vi "stimulate_and_record_async_daq.vi"(3 "SSH password":string, 4 "Transfer and Run Date Folder After Experiment":bool, 5 "SSH user name":string, 6 "Tags":string, 7 "Frames":i32, 8 "Convert Power to Voltage":bool, 9 "voltages/power":dbl[](array[numeric]), 10 "parameters":string[](array[string]), 11 "parameters headers":string[](array[string])) -> ()   [LabVIEW 2016]
uses:
  <vilib>/vision/driver/IMAQdx.llb/IMAQdx Acquisition Mode.ctl
  <vilib>/userdefined/High Color/IMAQdx.ctl
  <vilib>/vision/driver/IMAQdx.llb/IMAQdx Buffer Number Mode.ctl
  <vilib>/Utility/file.llb/Write To Spreadsheet File (DBL).vi
  <vilib>/Utility/file.llb/Write To Spreadsheet File (string).vi
  <vilib>/Utility/file.llb/Read From Spreadsheet File (string).vi
  <vilib>/vision/driver/NI_Vision_Acquisition_Software.lvlib
panel:
  out "DAC0 Voltage":dbl format="%.6f"
  out "error out 2":errorcluster
  out "Saved Buffer Number":u32
  out "ProcessFrameRate":dbl
  out "# elements in queue":i32
  out "CameraFrameRate":dbl
  out "Camera Buffer Number":u32
  out "Image":T1(plugin-control)
  out "JPEG Quality":dbl
  out "Save Directory":path
  in  "stop":bool
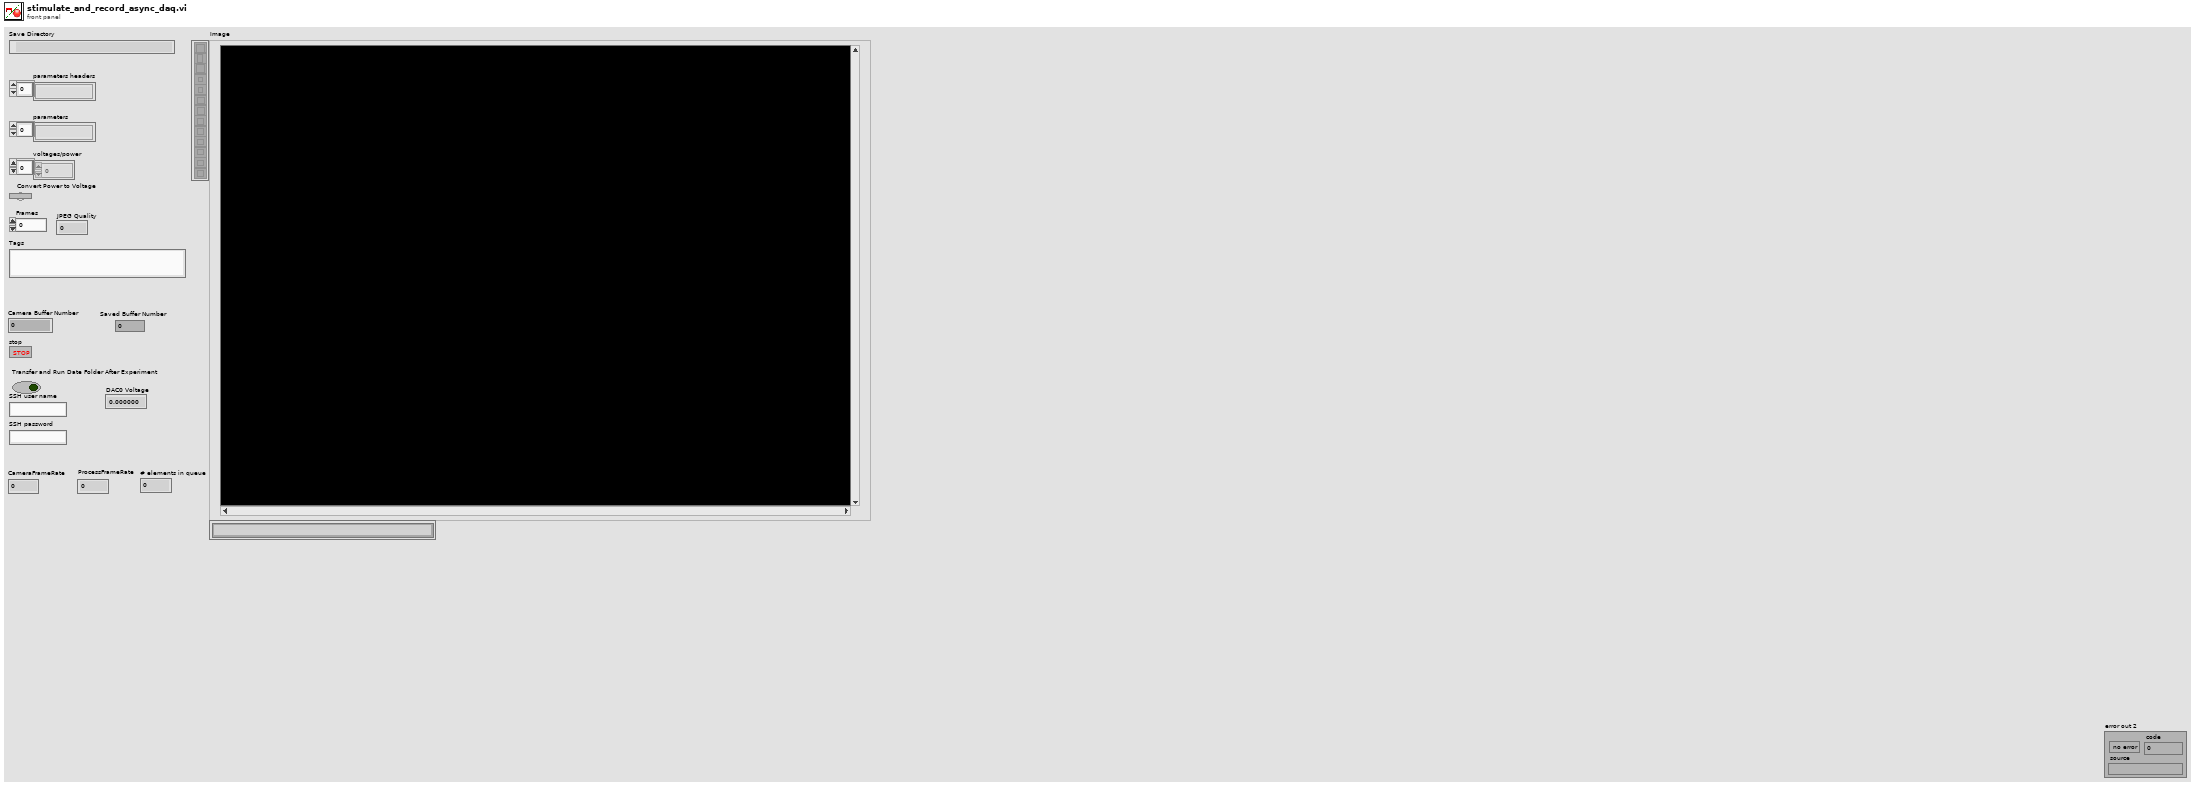
[diagram p1: front panel]
types:
  T1 = typedef "IMAQ Image.ctl" = refnum<image>
  T2 = typedef "IMAQdx.ctl" = refnum<k21>
  T3 = typedef "NI_Vision_Acquisition_Software.lvlib/IMAQdx Buffer Number Mode.ctl" = enum32{"Next", "Last", "Buffer Number", "Every", "Last New"}
  T4 = typedef "Image Type" = u32
  T5 = typedef "NI_Vision_Acquisition_Software.lvlib/IMAQdx Acquisition Mode.ctl" = enum32{"One Shot", "Continuous"}
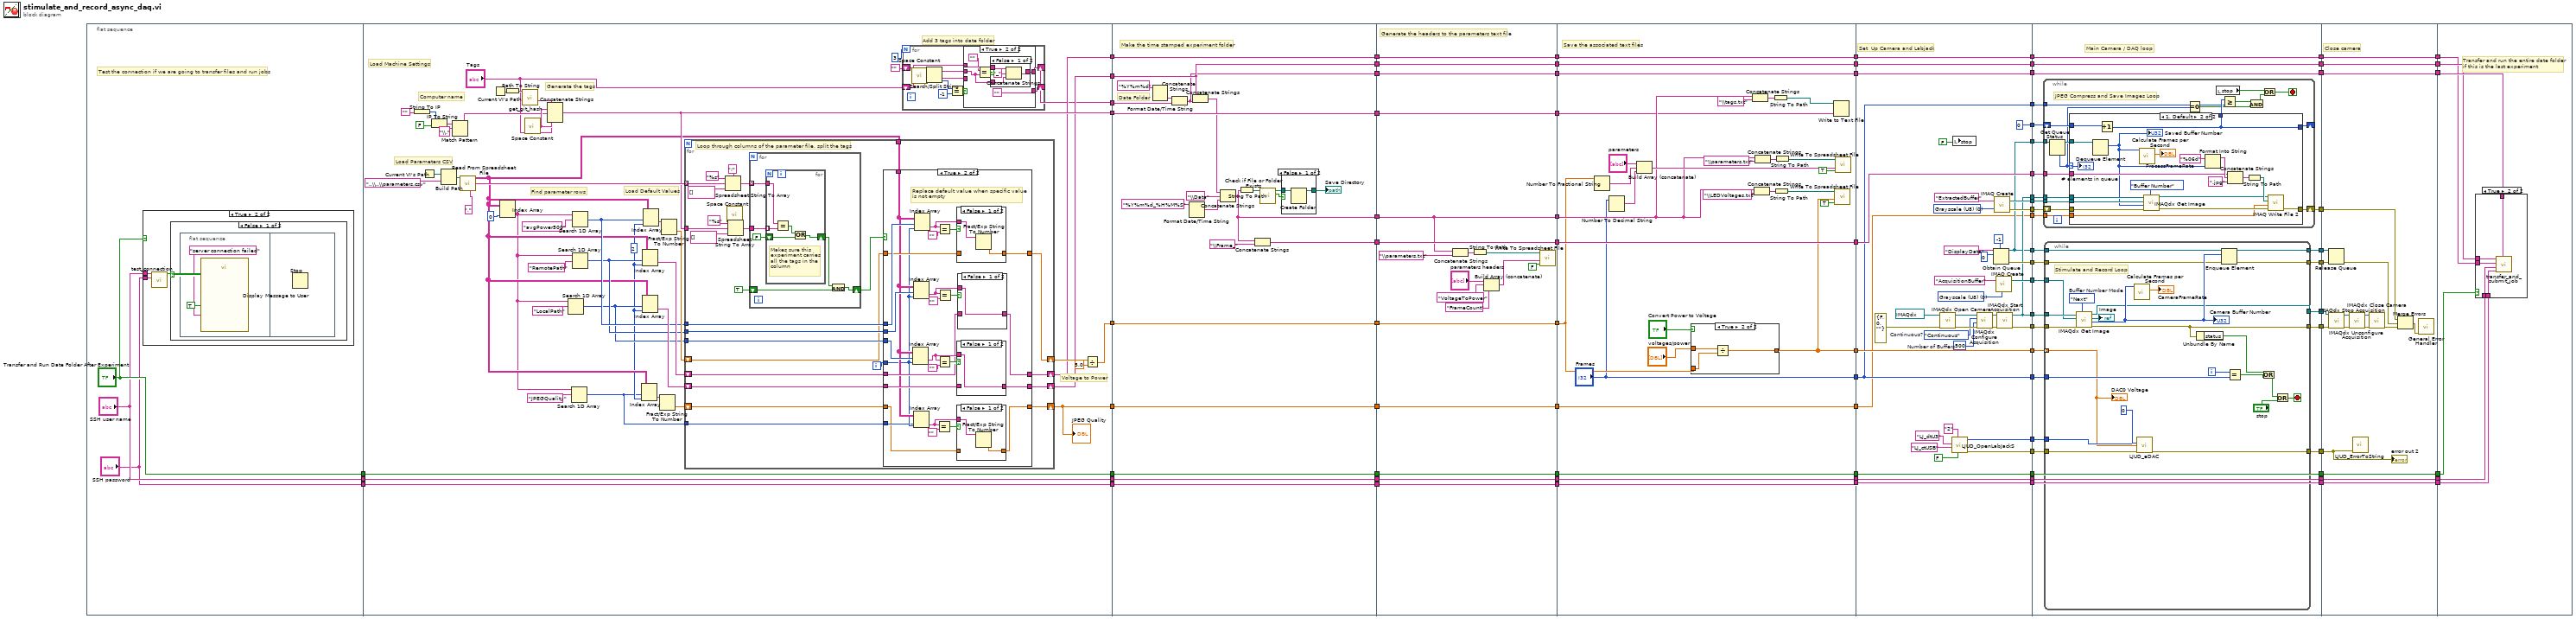
[diagram p0: block diagram]
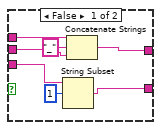
[diagram p4: hidden frame]
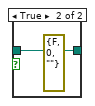
[diagram p11: hidden frame]
diagram:
  n1 = flat-sequence {
    tunnel: ["Transfer and Run Date Folder After Experiment"] -> w50
    tunnel: ["SSH user name"] -> w49
    tunnel: ["SSH password"] -> w48
    tunnel: [w132] -> w80
    tunnel: [w115] -> w79
    tunnel: [w106] -> w70
    tunnel: [w107] -> w69
    tunnel: w50 -> [w124]
    tunnel: w49 -> [w123]
    tunnel: w48 -> [w122]
    tunnel: [w124] -> w41
    tunnel: [w123] -> w34
    tunnel: [w122] -> w33
    tunnel: [w103] -> w26
    tunnel: [w94] -> w25
    tunnel: [w268] -> w64
    tunnel: [w267] -> w62
    tunnel: [w266] -> w60
    tunnel: [w265] -> w58
    tunnel: [w247] -> w56
    tunnel: [w249] -> w54
    tunnel: [w264] -> w52
    tunnel: w69 -> [w264]
    tunnel: w70 -> [w249]
    tunnel: w79 -> [w265]
    tunnel: w80 -> [w266]
    tunnel: [w256] -> w42
    tunnel: w41 -> [w256]
    tunnel: [w255] -> w35
    tunnel: w34 -> [w255]
    tunnel: w33 -> [w254]
    tunnel: [w254] -> w32
    tunnel: w26 -> [w250]
    tunnel: w25 -> [w246]
    tunnel: [w246] -> w22
    tunnel: w64 -> [w290]
    tunnel: [w290] -> w63
    tunnel: w62 -> [w276]
    tunnel: [w276] -> w61
    tunnel: w60 -> [w289]
    tunnel: [w289] -> w59
    tunnel: w58 -> [w288]
    tunnel: [w288] -> w57
    tunnel: w56 -> [w287]
    tunnel: [w287] -> w55
    tunnel: w54 -> [w286]
    tunnel: [w286] -> w53
    tunnel: w52 -> [w285]
    tunnel: [w285] -> w51
    tunnel: [w275] -> w43
    tunnel: w42 -> [w275]
    tunnel: [w274] -> w36
    tunnel: w35 -> [w274]
    tunnel: w32 -> [w273]
    tunnel: [w273] -> w31
    tunnel: [w272] -> w23
    tunnel: w22 -> [w272]
    tunnel: w63 -> [w318]
    tunnel: [w318] -> w85
    tunnel: [w301] -> w83
    tunnel: ["Frames"] -> w82
    tunnel: w61 -> [w310]
    tunnel: w59 -> [w297]
    tunnel: w57 -> [w292]
    tunnel: w55 -> [w306]
    tunnel: [w306] -> w75
    tunnel: [w305] -> w71
    tunnel: w53 -> [w305]
    tunnel: [w304] -> w65
    tunnel: w51 -> [w304]
    tunnel: [w295] -> w44
    tunnel: w43 -> [w295]
    tunnel: [w294] -> w37
    tunnel: w36 -> [w294]
    tunnel: w31 -> [w293]
    tunnel: [w293] -> w30
    tunnel: [w291] -> w24
    tunnel: w23 -> [w291]
    tunnel: w85 -> [w336]
    tunnel: [w364] -> w84
    tunnel: w83 -> [w364]
    tunnel: w82 -> [w335]
    tunnel: [w335] -> w81
    tunnel: [w363] -> w76
    tunnel: w75 -> [w363]
    tunnel: [w362] -> w72
    tunnel: w71 -> [w362]
    tunnel: [w361] -> w66
    tunnel: w65 -> [w361]
    tunnel: [w360] -> w45
    tunnel: w44 -> [w360]
    tunnel: [w359] -> w38
    tunnel: w37 -> [w359]
    tunnel: w30 -> [w358]
    tunnel: [w358] -> w29
    tunnel: w24 -> [w333]
    tunnel: [w342] -> w21
    tunnel: [w337] -> w20
    tunnel: [w341] -> w19
    tunnel: [w340] -> w18
    tunnel: [w334] -> w17
    tunnel: [w339] -> w14
    tunnel: [w338] -> w13
    tunnel: [w337] -> w12
    tunnel: [w336] -> w11
    tunnel: [w335] -> w10
    tunnel: [w334] -> w9
    tunnel: [w333] -> w8
    tunnel: [0] -> w5
    tunnel: [w326] -> w3
    tunnel: [w325] -> w2
    tunnel: w84 -> [w393]
    tunnel: w81 -> [w392]
    tunnel: [w391] -> w77
    tunnel: w76 -> [w391]
    tunnel: [w390] -> w73
    tunnel: w72 -> [w390]
    tunnel: [w389] -> w67
    tunnel: w66 -> [w389]
    tunnel: [w388] -> w46
    tunnel: w45 -> [w388]
    tunnel: [w387] -> w39
    tunnel: w38 -> [w387]
    tunnel: w29 -> [w386]
    tunnel: [w386] -> w28
    tunnel: w21 -> [w385]
    tunnel: w20 -> [w384]
    tunnel: w19 -> [w383]
    tunnel: w18 -> [w382]
    tunnel: w17 -> [w381]
    tunnel: [w380] -> w16
    tunnel: [w379] -> w15
    tunnel: w14 -> [w378]
    tunnel: w13 -> [w377]
    tunnel: w12 -> [w376]
    tunnel: w11 -> [w375]
    tunnel: w10 -> [w374]
    tunnel: w9 -> [w373]
    tunnel: w8 -> [w372]
    tunnel: [w369] -> w7
    tunnel: [w371] -> w6
    tunnel: w5 -> [w370]
    tunnel: [w368] -> w4
    tunnel: w3 -> [w367]
    tunnel: w2 -> [w366]
    tunnel: [w365] -> w1
    tunnel: [w476] -> w78
    tunnel: w77 -> [w476]
    tunnel: [w475] -> w74
    tunnel: w73 -> [w475]
    tunnel: [w474] -> w68
    tunnel: w67 -> [w474]
    tunnel: [w473] -> w47
    tunnel: w46 -> [w473]
    tunnel: [w472] -> w40
    tunnel: w39 -> [w472]
    tunnel: w28 -> [w471]
    tunnel: [w471] -> w27
    tunnel: w16 -> [w466]
    tunnel: w15 -> [w465]
    tunnel: w7 -> [w462]
    tunnel: w6 -> [w461]
    tunnel: w4 -> [w460]
    tunnel: w1 -> [w459]
    tunnel: w78 -> [w482]
    tunnel: w74 -> [w481]
    tunnel: w68 -> [w480]
    tunnel: w47 -> [w479]
    tunnel: w40 -> [w478]
    tunnel: w27 -> [w477]
    frame #0 {
      # "Test the connection if we are going to transfer files and run jobs"
      n2 = case shown="True" "Transfer and Run Date Folder After Experiment" {
        tunnel: "SSH password" -> [_ w91]
        tunnel: "SSH user name" -> [_ w89]
        frame False {
        }
        frame True {
          n3 = call "test_connection.vi"("Username"=w89, "Password"=w91) -> ("Connection Successful"=w90:bool)  [unwired: 7 in]
          n4 = case shown="False" w90 {
            frame False {
              n5 = flat-sequence {
                frame #0 {
                  n6 = call "Display Message to User"("Enable"=TRUE, "Message"="server connection failed") -> ()  [unwired: 8 in, 2 out]
                }
                frame #1 {
                  n7 = Stop() -> ()  [unwired: 1 in]
                }
              }
            }
            frame True {
            }
          }
        }
      }
    }
    frame #1 {
      w97 = 2
      # "Add 3 tags into date folder"
      # "Generate the tags"
      # "Find parameter rows"
      # "Load Default Values"
      # "Voltage to Power"
      # "Load Parameters CSV"
      # "Computer name"
      # "Load Machine Settings"
      n8 = String To IP(1:"") -> (0:w140:u32)
      n9 = Current VI's Path() -> (path=w135:path)
      n10 = IP To String(1:FALSE, 2:w140) -> (0:w137:string)
      n11 = Build Path(base path=w135, name or relative path="..\\..\\parameters.csv") -> (appended path=w126:path)
      n12 = Match Pattern(string=w137, regular expression="\\.") -> (before substring=w117:string)  [unwired: 1 in, 3 out]
      n13 = call-poly <vilib>:"Read From Spreadsheet File.vi"("delimiter (\\t)"=",", "file path (dialog if empty)"=w126) -> ("first row"=w116:string[], "all rows"=w99:string[][])  [unwired: 5 in, 3 out]
      n14 = Current VI's Path() -> (path=w119:path)
      n15 = Index Array(array=w99, index (col)=0) -> (element=w98:string[])  [unwired: 1 in]
      n16 = Path To String(path=w119) -> (string=w118:string)
      n17 = call "get_git_hash.vi"("VI folder"=w118) -> ("github hash"=w121:string)  [unwired: 10 in]
      n18 = call <vilib>:"Space Constant.vi"() -> ("String"=w120:string)
      n19 = Concatenate Strings(w121, w120, w117, w120, "Tags") -> (w115:string)
      n20 = Search 1D Array(1D array=w98, element="LocalPath") -> (index of element=w109:i32)  [unwired: 1 in]
      n21 = Search 1D Array(1D array=w98, element="JPEGQuality") -> (index of element=w95:i32)  [unwired: 1 in]
      n22 = Search 1D Array(1D array=w98, element="RemotePath") -> (index of element=w110:i32)  [unwired: 1 in]
      n23 = Search 1D Array(1D array=w98, element="avgPower500") -> (index of element=w111:i32)  [unwired: 1 in]
      n24 = Index Array(array=w99, index (row)=w95, index (col)=w97) -> (element=w100:string)
      n25 = Index Array(array=w99, index (row)=w110, index (col)=w97) -> (element=w113:string)
      n26 = Index Array(array=w99, index (row)=w109, index (col)=w97) -> (element=w112:string)
      n27 = Index Array(array=w99, index (row)=w111, index (col)=w97) -> (element=w128:string)
      n28 = Fract/Exp String To Number(string=w100) -> (number=w96:dbl)  [unwired: 3 in, 1 out]
      n29 = Fract/Exp String To Number(string=w128) -> (number=w114:dbl)  [unwired: 3 in, 1 out]
      n30 = for {
        tunnel: w116 -> [w194] mode=indexing
        tunnel: w115 -> [w186]
        tunnel: w111 -> [w181]
        tunnel: w110 -> [w180]
        tunnel: w109 -> [w179]
        tunnel: w99 -> [w184]
        shift-right: [w176] -> w108
        shift-left: w114 -> [w177]
        shift-right: [w173] -> w107
        shift-left: w113 -> [w174]
        shift-right: [w172] -> w106
        shift-left: w112 -> [w175]
        shift-right: [w169] -> w94
        shift-left: w96 -> [w171]
        tunnel: w95 -> [w170]
        i -> [w178]
        # "Loop through columns of the parameter file, split the tags"
        n31 = Spreadsheet String To Array(delimiter (Tab)=";", format string="%s", spreadsheet string=w194, array type (2D Dbl)=string[] []) -> (array=w190:string[])
        n32 = call <vilib>:"Space Constant.vi"() -> ("String"=w188:string)
        n33 = Spreadsheet String To Array(delimiter (Tab)=w188, format string="%s", spreadsheet string=w186, array type (2D Dbl)=string[] []) -> (array=w185:string[])
        n34 = for {
          tunnel: w190 -> [w240] mode=indexing
          tunnel: w185 -> [w239]
          shift-right: [w237] -> w182
          shift-left: TRUE -> [w235]
          n35 = for {
            tunnel: w240 -> [w245]
            tunnel: w239 -> [w244] mode=indexing
            shift-right: [w241] -> w236
            shift-left: FALSE -> [w242]
            # "Makes sure this\nexperiment carries\nall the tags in the\ncolumn"
            n36 = Equal?(x=w245, y=w244) -> (x = y?=w243:bool)
            n37 = Or(x=w243, y=w242) -> (x .or. y?=w241:bool)
          }
          n38 = And(x=w236, y=w235) -> (x .and. y?=w237:bool)
        }
        n39 = case shown="True" w182 {
          tunnel: w177 -> [w198 w219]
          tunnel: [w198 w218] -> w176
          tunnel: w181 -> [_ w224]
          tunnel: w180 -> [_ w223]
          tunnel: w179 -> [_ w222]
          tunnel: w178 -> [_ w201]
          tunnel: w184 -> [_ w202]
          tunnel: [w197 w208] -> w173
          tunnel: [w196 w210] -> w172
          tunnel: w175 -> [w196 w209]
          tunnel: w174 -> [w197 w207]
          tunnel: w171 -> [w195 w199]
          tunnel: w170 -> [_ w200]
          tunnel: [w195 w203] -> w169
          frame False {
          }
          frame True {
            # "Replace default value when specific value\nis not empty"
            n40 = Index Array(array=w202, index (row)=w222, index (col)=w201) -> (element=w211:string)
            n41 = Index Array(array=w202, index (row)=w223, index (col)=w201) -> (element=w214:string)
            n42 = Index Array(array=w202, index (row)=w200, index (col)=w201) -> (element=w204:string)
            n43 = Index Array(array=w202, index (row)=w224, index (col)=w201) -> (element=w217:string)
            n44 = Equal?(x=w204, y="") -> (x = y?=w205:bool)
            n45 = Equal?(x=w217, y="") -> (x = y?=w220:bool)
            n46 = Equal?(x=w211, y="") -> (x = y?=w212:bool)
            n47 = Equal?(x=w214, y="") -> (x = y?=w215:bool)
            n48 = case shown="False" w205 {
              tunnel: w199 -> [_ w227]
              tunnel: [w226 w227] -> w203
              tunnel: w204 -> [w225 _]
              frame False {
                n49 = Fract/Exp String To Number(string=w225) -> (number=w226:dbl)  [unwired: 3 in, 1 out]
              }
              frame True {
              }
            }
            n50 = case shown="False" w220 {
              tunnel: w219 -> [_ w234]
              tunnel: [w233 w234] -> w218
              tunnel: w217 -> [w232 _]
              frame False {
                n51 = Fract/Exp String To Number(string=w232) -> (number=w233:dbl)  [unwired: 3 in, 1 out]
              }
              frame True {
              }
            }
            n52 = case shown="False" w212 {
              tunnel: w211 -> [w228 _]
              tunnel: [w228 w229] -> w210
              tunnel: w209 -> [_ w229]
              frame False {
              }
              frame True {
              }
            }
            n53 = case shown="False" w215 {
              tunnel: w214 -> [w230 _]
              tunnel: [w230 w231] -> w208
              tunnel: w207 -> [_ w231]
              frame False {
              }
              frame True {
              }
            }
          }
        }
      }
      "JPEG Quality" <- w94
      n54 = for {
        N: 3 -> [_]
        shift-right: [w141] -> _
        shift-left: "Tags" -> [w150]
        shift-right: [w143] -> w103
        shift-left: "" -> [w148]
        n55 = call <vilib>:"Space Constant.vi"() -> ("String"=w149:string)
        n56 = Search/Split String(string=w150, search string/char (-)=w149) -> (substring before match=w147:string, match + rest of string=w146:string, offset of match=w145:i32)  [unwired: 1 in]
        n57 = Equal?(x=w145, y=-1) -> (x = y?=w142:bool)
        n58 = case shown="True" w142 {
          tunnel: w148 -> [w151 w161]
          tunnel: w147 -> [w152 w158]
          tunnel: w146 -> [w153 _]
          tunnel: [w155 ""] -> w141
          tunnel: [w154 w160] -> w143
          frame False {
            n59 = String Subset(string=w153, offset (0)=1) -> (substring=w155:string)  [unwired: 1 in]
            n60 = Concatenate Strings(w151, "_", w152) -> (w154:string)
          }
          frame True {
            n61 = Equal?(x="", y=w158) -> (x = y?=w162:bool)
            n62 = case shown="False" w162 {
              tunnel: w161 -> [w165 w168]
              tunnel: [w166 w168] -> w160
              tunnel: w158 -> [w164 _]
              frame False {
                n63 = Concatenate Strings(w165, "_", w164) -> (w166:string)
              }
              frame True {
              }
            }
          }
        }
      }
      n64 = Divide(x=w108, y=5.0) -> (x/y=w132:dbl)
    }
    frame #2 {
      # "Make the time stamped experiment folder"
      # "Date Folder"
      n65 = Format Date/Time String(time format string (%c)="%Y%m%d") -> (date/time string=w251:string)  [unwired: 2 in]
      n66 = Concatenate Strings(w251, w250) -> (w247:string)
      n67 = Format Date/Time String(time format string (%c)="%Y%m%d_%H%M%S") -> (date/time string=w253:string)  [unwired: 2 in]
      n68 = Concatenate Strings(w249, w247) -> (w248:string)
      n69 = Concatenate Strings(w248, "\\Data", w253) -> (w267:string)
      n70 = String To Path(string=w267) -> (path=w259:path)
      n71 = Concatenate Strings(w267, "\\Frame_") -> (w268:string)
      n72 = call <vilib>:"Check if File or Folder Exists.vi"("path"=w259) -> ("file or folder exists?"=w262:bool, "dup path"=w261:path)  [unwired: 8 in, 1 out]
      n73 = case shown="False" w262 {
        tunnel: [w269 w271] -> w258
        tunnel: w261 -> [w270 w271]
        frame False {
          n74 = Create Folder(path (use dialog)=w270) -> (created path=w269:path)  [unwired: 2 in, 2 out]
        }
        frame True {
          (unwired) errorcluster {"status"=FALSE, "code"=0, "source"=""} ("error out")
        }
      }
      "Save Directory" <- w258
    }
    frame #3 {
      # "Generate the headers to the parameters text file"
      n75 = Concatenate Strings(w276, "\\parameters.txt") -> (w284:string)
      n76 = String To Path(string=w284) -> (path=w283:path)
      n77 = Build Array (concatenate)("parameters headers", "VoltageToPower", "FrameCount") -> (w280:string[])
      n78 = call-poly <vilib>:"Write To Spreadsheet File.vi"("append to file? (new file:F)"=FALSE, "1D data"=w280, "file path (dialog if empty)"=w283) -> ()  [unwired: 5 in, 1 out]
    }
    frame #4 {
      # "Save the associated text files"
      n79 = Number To Fractional String(number=w297) -> (F-format string=w298:string)  [unwired: 3 in]
      n80 = Number To Decimal String(number="Frames") -> (decimal integer string=w299:string)  [unwired: 1 in]
      n81 = Build Array (concatenate)("parameters", w298, w299) -> (w311:string[])
      n82 = case shown="True" "Convert Power to Voltage" {
        tunnel: "voltages/power" -> [w321 w324]
        tunnel: [w321 w322] -> w301
        tunnel: w297 -> [_ w323]
        frame False {
        }
        frame True {
          n83 = Divide(x=w324, y=w323) -> (x/y=w322:dbl[])
        }
      }
      n84 = Concatenate Strings(w310, "\\tags.txt") -> (w308:string)
      n85 = Concatenate Strings(w310, "\\LEDVoltages.txt") -> (w320:string)
      n86 = Concatenate Strings(w310, "\\parameters.txt") -> (w315:string)
      n87 = String To Path(string=w308) -> (path=w307:path)
      n88 = String To Path(string=w320) -> (path=w319:path)
      n89 = String To Path(string=w315) -> (path=w314:path)
      n90 = Write to Text File(file (use dialog)=w307, text=w292) -> ()  [unwired: 2 in, 3 out]
      n91 = call-poly <vilib>:"Write To Spreadsheet File.vi"("append to file? (new file:F)"=TRUE, "1D data"=w301, "file path (dialog if empty)"=w319) -> ()  [unwired: 5 in, 1 out]
      n92 = call-poly <vilib>:"Write To Spreadsheet File.vi"("append to file? (new file:F)"=TRUE, "1D data"=w311, "file path (dialog if empty)"=w314) -> ()  [unwired: 5 in, 1 out]
    }
    frame #5 {
      w345 = T4 0 items=["Grayscale (U8)", "Grayscale (I16)", "Grayscale (SGL)", "Complex (CSG)", "RGB (U32)", "HSL (U32)", "RGB (U64)"] ("Image Type")
      w354 = T4 0 items=["Grayscale (U8)", "Grayscale (I16)", "Grayscale (SGL)", "Complex (CSG)", "RGB (U32)", "HSL (U32)", "RGB (U64)"] ("Image Type")
      w355 = u32 500  # Number of Buffers
      w351 = IMAQdx_Acquisition_Mode."Continuous"  # Continuous?
      # "Set  Up Camera and Labjack"
      n93 = call <vilib>:"IMAQdx Open Camera.vi"("error in"=errorcluster {"status"=FALSE, "code"=0, "source"=""}, "Session In"=T2 "cam0") -> ("error out"=w356:errorcluster, "Session Out"=w357:T2)  [unwired: 8 in]
      n94 = call "LJUD_OpenLabJackS.vi"("FirstFound"=FALSE, "Address"="2", "ConnectionType"="LJ_ctUSB", "DeviceType"="LJ_dtU3") -> ("error out"=w325:errorcluster, "Handle"=w326:i32)  [unwired: 5 in, 1 out]
      n95 = local write "stop"(FALSE) -> ()
      n96 = call <vilib>:"IMAQdx Configure Acquisition.vi"("error in"=w356, "Number of Buffers"=w355, "Continuous?"=w351, "Session In"=w357) -> ("error out"=w352:errorcluster, "Session Out"=w350:T2)  [unwired: 6 in]
      n97 = Obtain Queue(max queue size (-1, unlimited)=-1, name (unnamed)="DisplayData", element data type=u32 0) -> (queue out=w334:refnum<queue>, error out=w340:errorcluster)  [unwired: 2 in, 1 out]
      n98 = call "IMAQ Create"("Image Name"="ExtractedBuffer", "Image Type"=w345) -> ("New Image"=w338:T1, "error out"=w339:errorcluster)  [unwired: 3 in]
      n99 = call "IMAQ Create"("Image Name"="AcquisitionBuffer", "Image Type"=w354) -> ("New Image"=w341:T1)  [unwired: 3 in, 1 out]
      n100 = call <vilib>:"IMAQdx Start Acquisition.vi"("error in"=w352, "Session In"=w350) -> ("error out"=w342:errorcluster, "Session Out"=w337:T2)  [unwired: 8 in]
    }
    frame #6 {
      # "Main Camera / DAQ loop"
      n101 = while {
        tunnel: w373 -> [w411]
        tunnel: w377 -> [w409]
        tunnel: w376 -> [w408]
        tunnel: w375 -> [w406]
        shift-right: [w405] -> w371
        shift-left: w378 -> [w407]
        tunnel: w374 -> [w398]
        tunnel: w372 -> [w403]
        shift-right: [w400] -> _
        shift-left: w370 -> [w401]
        stop <- w404 stop-if-true
        # "JPEG Compress and Save Images Loop"
        n102 = Get Queue Status(queue=w411) -> (queue out=w410:refnum<queue>, # elements in queue=w394:i32)  [unwired: 2 in, 6 out]
        n103 = case shown="1, Default" w394 {
          selector: w394 -> [_ w432]
          tunnel: w410 -> [_ w430]
          tunnel: w409 -> [_ w429]
          tunnel: w408 -> [_ w428]
          tunnel: w407 -> [w413 w427]
          tunnel: w406 -> [_ w421]
          tunnel: [w413 w417] -> w405
          tunnel: w403 -> [_ w416]
          tunnel: w401 -> [w412 w415]
          tunnel: [w412 w414] -> w400
          tunnel: [w412 w414] -> w399
          frame 0 {
          }
          frame 1, Default {
            n104 = Dequeue Element(queue=w430) -> (element=w418:u32)  [unwired: 2 in, 3 out]
            "Saved Buffer Number" <- w418
            n105 = Increment(x=w415) -> (x+1=w414:i32)
            n106 = call <vilib>:"Calculate Frames per Second.vi"("Buffer Number"=w418) -> ("Processed Frames/s"=→"ProcessFrameRate":dbl)  [unwired: 8 in, 2 out]
            n107 = call <vilib>:"IMAQdx Get Image.vi"("Buffer Number Mode (Next)"=IMAQdx_Buffer_Number_Mode."Buffer Number", "error in"=w427, "Buffer Number In"=w418, "Image In"=w429, "Session In"=w428) -> ("error out"=w419:errorcluster, "Image Out"=w420:T1)  [unwired: 3 in, 2 out]
            n108 = Format Into String(format string="%06d" ("string"), w418) -> (resulting string=w423:string)  [unwired: 2 in, 1 out]
            n109 = Concatenate Strings(w421, w423, ".jpg" ("string")) -> (w425:string)
            n110 = String To Path(string=w425) -> (path=w424:path)
            n111 = call-poly "IMAQ Write File 2"("error in (no error)"=w419, "Image Quality"=w416, "File Path"=w424, "Image"=w420) -> ("error out"=w417:errorcluster)  [unwired: 6 in, 1 out]
            "# elements in queue" <- w432
          }
        }
        n112 = Equal To 0?(x=w394) -> (x = 0?=w395:bool)
        n113 = local read "stop"() -> (w402:bool)
        n114 = Greater Or Equal?(x=w399, y=w398) -> (x >= y?=w397:bool)
        n115 = And(x=w397, y=w395) -> (x .and. y?=w396:bool)
        n116 = Or(x=w402, y=w396) -> (x .or. y?=w404:bool)
      }
      n117 = while {
        tunnel: w393 -> [w434] mode=indexing
        tunnel: w392 -> [w455]
        tunnel: w385 -> [w450]
        tunnel: w384 -> [w449]
        tunnel: w383 -> [w448]
        tunnel: w382 -> [w447]
        tunnel: w381 -> [w446]
        tunnel: [w443] -> w368
        tunnel: [w442] -> w369
        tunnel: [w441] -> w380
        tunnel: [w440] -> w379
        tunnel: w367 -> [w437]
        tunnel: w366 -> [w436]
        tunnel: [w435] -> w365
        i -> [w456]
        stop <- w458 stop-if-true
        w454 = IMAQdx_Buffer_Number_Mode."Next"  # Buffer Number Mode
        # "Stimulate and Record Loop"
        n118 = call <vilib>:"IMAQdx Get Image.vi"("Buffer Number Mode (Next)"=w454, "error in"=w450, "Image In"=w448, "Session In"=w449) -> ("error out"=w440:errorcluster, "Buffer Number Out"=w451:u32, "Image Out"=→"Image":T1, "Session Out"=w441:T2)  [unwired: 4 in]
        "Camera Buffer Number" <- w451
        n119 = call <vilib>:"Calculate Frames per Second.vi"("Buffer Number"=w451) -> ("Processed Frames/s"=→"CameraFrameRate":dbl)  [unwired: 8 in, 2 out]
        n120 = call "LJUD_eDAC.vi"("Handle In"=w437, "Channel"=0, "Voltage"=w434, "error in"=w436) -> ("error out"=w435:errorcluster)  [unwired: 10 in, 1 out]
        n121 = Unbundle By Name(w440) -> ("status"=w445:bool)
        n122 = Enqueue Element(queue=w446, element=w451, error in (no error)=w447) -> (queue out=w443:refnum<queue>, error out=w442:errorcluster)  [unwired: 1 in, 1 out]
        n123 = Equal?(x=w456, y=w455) -> (x = y?=w439:bool)
        n124 = Or(x=w445, y=w439) -> (x .or. y?=w444:bool)
        n125 = Or(x=w444, y="stop") -> (x .or. y?=w458:bool)
        "DAC0 Voltage" <- w434
      }
    }
    frame #7 {
      # "Close camera"
      n126 = Release Queue(queue=w460) -> ()  [unwired: 2 in, 3 out]
      n127 = call <vilib>:"IMAQdx Stop Acquisition.vi"("error in"=w465, "Session In"=w466) -> ("error out"=w467:errorcluster, "Session Out"=w468:T2)  [unwired: 8 in]
      n128 = call <vilib>:"IMAQdx Unconfigure Acquisition.vi"("error in"=w467, "Session In"=w468) -> ("error out"=w470:errorcluster, "Session Out"=w469:T2)  [unwired: 8 in]
      n129 = call "LJUD_ErrorToString.vi"("error in"=w459) -> ()  [unwired: 10 in, 1 out]
      n130 = call <vilib>:"IMAQdx Close Camera.vi"("error in"=w470, "Session In"=w469) -> ("error out"=w463:errorcluster)  [unwired: 9 in]
      n131 = Merge Errors(w461, w462, w463) -> (w464:errorcluster)
      n132 = call <vilib>:"General Error Handler.vi"("error in (no error)"=w464) -> ()  [unwired: 10 in, 5 out]
      "error out 2" <- w459
    }
    frame #8 {
      # "Transfer and run the entire date folder\nif this is the last experiment"
      n133 = case shown="True" w479 {
        tunnel: w482 -> [_ w487]
        tunnel: w481 -> [_ w486]
        tunnel: w480 -> [_ w485]
        tunnel: w478 -> [_ w484]
        tunnel: w477 -> [_ w483]
        frame False {
        }
        frame True {
          n134 = call "transfer_and_submit_job.vi"("Date Folder"=w487, "Password"=w483, "Username"=w484, "Remote Data Directory"=w485, "Local Data Directory"=w486) -> ()  [unwired: 7 in]
        }
      }
    }
  }
